vi "dtAppMain.vi"() -> ()   [LabVIEW 2016]
doc: "Top-level application."
uses:
  Typedefs/ContextID.ctl
  ContextIDFactory/ContextIDFactory.lvclass
  ContextThisComponent/ContextThisComponent.lvclass
  home/andres/ct_cmpuserevents/ComponentTemplateCore/ComponentModel/ComponentModel/Context/Context.lvclass
  InvokerThisComponent/InvokerThisComponent.lvclass
  home/andres/ct_cmpuserevents/ComponentTemplateCore/ComponentModel/ComponentModel/Invoker/Invoker.lvclass
  CommandFactory/CommandFactory.lvclass
  StateFactory/StateFactory.lvclass
  home/andres/ct_cmpuserevents/IStateFactory/IStateFactory.lvclass
  Model/Model/Model.lvclass
  home/andres/ct_cmpuserevents/IModel/IModel.lvclass
  PubSubDataEvent/PubSubDataEvent.lvclass
  MiddlewareSALThisComponent/MiddlewareSALThisComponent.lvclass
  home/andres/ct_cmpuserevents/ComponentTemplateCore/ComponentModel/ComponentModel/Middleware/Middleware.lvclass
  MiddlewareSALThisComponent/ProgrammaticInitialization/ProgrammaticInitialization.lvclass
  ComponentTemplateCore/ComponentModel/ComponentModel/UserEventBasedController/UserEventBasedController.lvclass
  home/andres/ct_cmpuserevents/ComponentTemplateCore/ComponentModel/ComponentModel/Controller/Controller.lvclass
  Typedefs/CommandValue.ctl
  ComponentTemplateCore/ComponentModel/ComponentModelRT/LoopTimer/LoopTimer/LoopTimer.lvclass
  home/andres/ct_cmpuserevents/ComponentTemplateCore/ComponentModel/ComponentModelRT/LoopTimer/ILoopTimer/ILoopTimer.lvclass
  ComponentTemplateCore/ComponentModel/ComponentModel/DTTLListener/DTTLListener.lvclass
  home/andres/ct_cmpuserevents/ComponentTemplateCore/ComponentModel/ComponentModel/TimedLoopListener/TimedLoopListener.lvclass
  Model/Target/WindowsTarget/WindowsTarget.lvclass
  home/andres/ct_cmpuserevents/Model/Target/Target/Target.lvclass
  ComponentTemplateCore/ComponentModel/ComponentModel/Heartbeat/Heartbeat/Heartbeat.lvclass
  home/andres/ct_cmpuserevents/ComponentTemplateCore/ComponentModel/ComponentModel/Heartbeat/IHeartbeat/IHeartbeat.lvclass
  ComponentTemplateCore/ComponentModel/ComponentModel/Rendezvous/Rendezvous.lvclass
  ComponentTemplateCore/ComponentModel/ComponentModel/CommandEvent/CommandEvent.lvclass
  ComponentTemplateCore/ComponentModel/ComponentModel/MiddlewareProcessEvent/MiddlewareProcessEvent.lvclass
  Model/Model/Model.lvclass/Model.ctl
  Typedefs/StateValue.ctl
  ts_sallv_exa/DataTypes/logevent_SummaryState.ctl
  ComponentTemplateCore/ComponentModel/ComponentModel/UserEventBasedController/UserEventBasedController.lvclass/UserEventBasedController.ctl
  ComponentTemplateCore/ComponentModel/ComponentModel/Middleware/Middleware.lvclass/Middleware.ctl
  ComponentTemplateCore/Application/AppDT/AppDT.lvclass
  ComponentTemplateCore/Application/AppDT/AppDT.lvclass/AppDT.ctl
  Typedefs/EXATypedefs.lvlib
  ComponentTemplateCore/ComponentModel/ComponentModel/Middleware/Middleware.lvclass
  ts_sallv_exa/SALLV_EXA.lvlib
  ComponentTemplateCore/ComponentModel/ComponentModel/ConfigurationFileReader/ConfigurationFileReader.lvclass
panel:
  out "error out":errorcluster
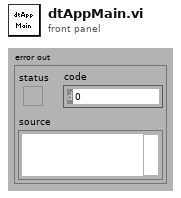
[diagram p1: front panel]
types:
  T1 = typedef "EXATypedefs.lvlib/ContextID.ctl" = enum16{"ExA"}
  T2 = typedef "EXATypedefs.lvlib/CommandValue.ctl" = enum16{"Disable", "Enable", "Exit", "GoToStandby", "OnHeartbeat", "OnIncomingMessagingError", "OnInterrupt", "Start"}
  T3 = typedef "SALLV_EXA.lvlib/logevent_SummaryState.ctl" = cluster{"summaryState":enum16{"", " OfflineState", "StandbyState", "DisabledState", "EnabledState", "FaultState"}, "priority":i32}
  T4 = typedef "EXATypedefs.lvlib/StateValue.ctl" = enum16{"", " DisabledState", "EnabledState", "FaultState", "OfflineState", "StandbyState"}
  T5 = typedef "ConfigurationTypedefs.lvlib/SALVisSettings.ctl" = cluster{"Subsystem":string, "SAL Vis Path":path, "Events":T6, "Telemetry":T7, "Commands":T8}
  T6 = typedef "ProgrammaticInitialization.lvclass/evntsToSubscribeView.ctl" = string[]
  T7 = typedef "ProgrammaticInitialization.lvclass/tlmtryToSubscribeView.ctl" = string[]
  T8 = typedef "ProgrammaticInitialization.lvclass/cmdsToSubscribeDL.ctl" = string[]
  T9 = enum32{"invalid app kind", "Development System", "Run Time System", "Student Edition", "Embedded LabVIEW", "Evaluation", "Custom"}
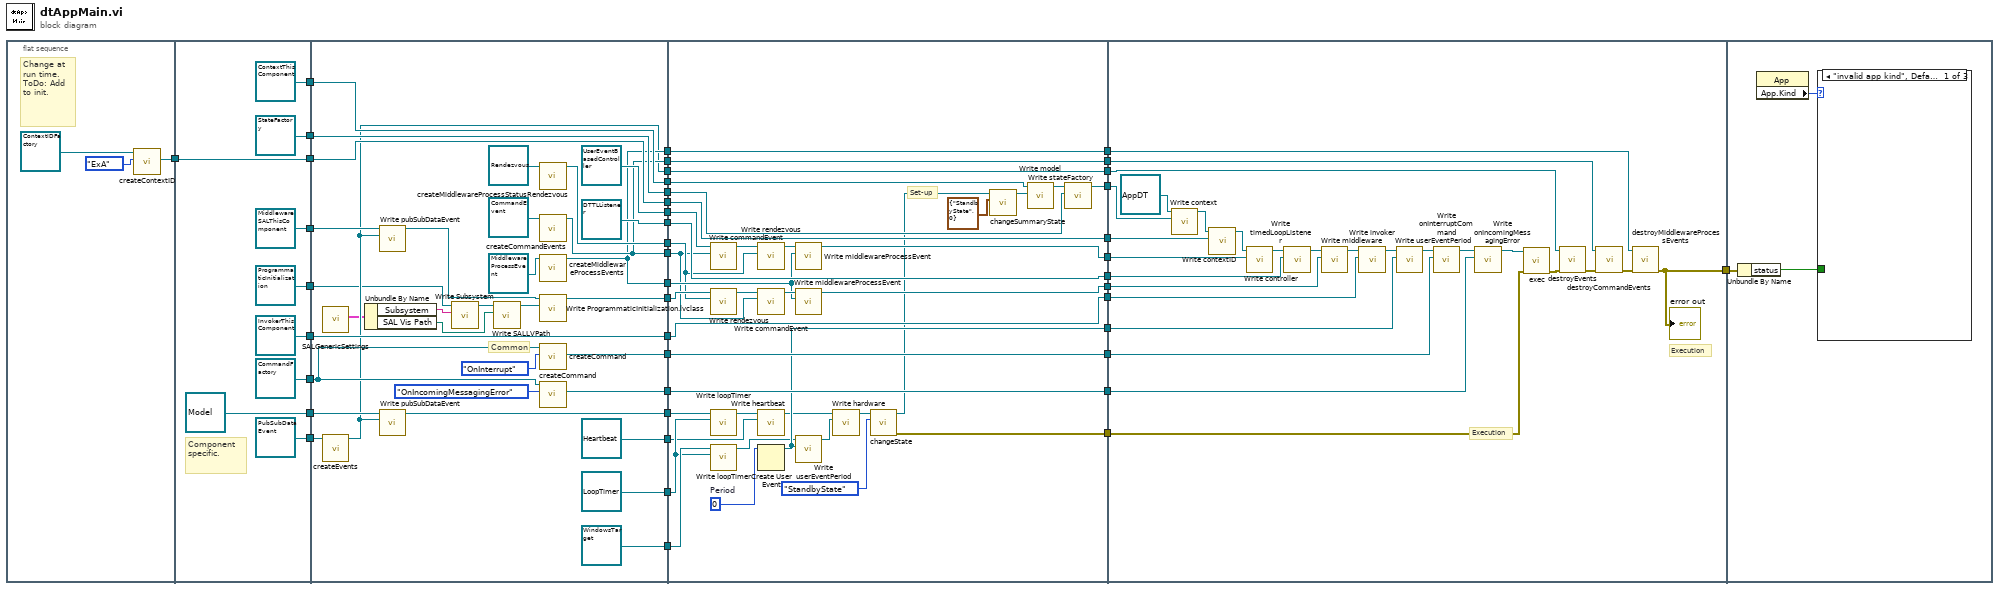
[diagram p0: block diagram]
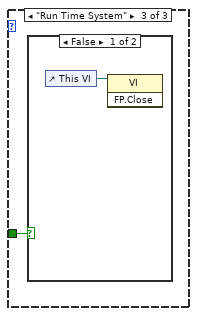
[diagram p3: hidden frame]
diagram:
  n1 = flat-sequence {
    tunnel: [w45] -> w36
    tunnel: [w53] -> w39
    tunnel: [refnum<class "ContextThisComponent.lvclass"> refnum ("ConcreteContext.lvlib:ConcreteContext1.lvclass")] -> w38
    tunnel: [refnum<class "InvokerThisComponent.lvclass"> refnum ("InvokerThisComponent.lvclass")] -> w37
    tunnel: w36 -> [w53]
    tunnel: [refnum<class "CommandFactory.lvclass"> refnum ("CommandFactory.lvclass")] -> w27
    tunnel: [refnum<class "StateFactory.lvclass"> refnum ("ConcreteStateFactory.lvlib:ConcreteStateFactory.lvclass")] -> w25
    tunnel: [refnum<class "Model.lvclass"> refnum ("ConcreteModel.lvclass")] -> w23
    tunnel: [refnum<class "MiddlewareSALThisComponent.lvclass"> refnum ("MiddlewareSALThisComponent.lvclass")] -> w14
    tunnel: [refnum<class "PubSubDataEvent.lvclass"> refnum ("pubSubDataEvent")] -> w13
    tunnel: [refnum<class "ProgrammaticInitialization.lvclass"> refnum ("ProgrammaticInitialization.lvclass")] -> w1
    tunnel: [w87] -> w43
    tunnel: [w86] -> w42
    tunnel: [refnum<class "UserEventBasedController.lvclass"> refnum ("UserEventBasedController in")] -> w41
    tunnel: [w85] -> w40
    tunnel: w39 -> [w87]
    tunnel: w38 -> [w86]
    tunnel: w37 -> [w85]
    tunnel: [refnum<class "DTTLListener.lvclass"> refnum ("DTTLListener.lvclass")] -> w30
    tunnel: [w84] -> w28
    tunnel: w27 -> [w80]
    tunnel: [w83] -> w26
    tunnel: w25 -> [w83]
    tunnel: [w66] -> w24
    tunnel: w23 -> [w67]
    tunnel: [refnum<class "LoopTimer.lvclass"> refnum ("ComponentModelRT.lvlib:LoopTimer.lvclass")] -> w22
    tunnel: [w78] -> w19
    tunnel: [refnum<class "WindowsTarget.lvclass"> refnum ("WindowsTarget.lvclass")] -> w17
    tunnel: [refnum<class "Heartbeat.lvclass"> refnum ("Heartbeat.lvclass")] -> w15
    tunnel: w14 -> [w65]
    tunnel: w13 -> [w74]
    tunnel: [w62] -> w12
    tunnel: [w70] -> w11
    tunnel: [w69] -> w10
    tunnel: [w68] -> w9
    tunnel: [w64] -> w6
    tunnel: [w69] -> w4
    tunnel: [w68] -> w2
    tunnel: w1 -> [w61]
    tunnel: w43 -> [w127]
    tunnel: w42 -> [w120]
    tunnel: w41 -> [w101]
    tunnel: w40 -> [w126]
    tunnel: [w127] -> w35
    tunnel: [w126] -> w34
    tunnel: [w97] -> w33
    tunnel: [w114] -> w32
    tunnel: [w125] -> w31
    tunnel: w30 -> [w125]
    tunnel: [w124] -> w29
    tunnel: w28 -> [w124]
    tunnel: w26 -> [w122]
    tunnel: w24 -> [w116]
    tunnel: w22 -> [w111]
    tunnel: [w121] -> w21
    tunnel: [w119] -> w20
    tunnel: w19 -> [w119]
    tunnel: [w90] -> w18
    tunnel: w17 -> [w115]
    tunnel: w15 -> [w108]
    tunnel: w12 -> [w107]
    tunnel: w11 -> [w102]
    tunnel: w10 -> [w100]
    tunnel: w9 -> [w103]
    tunnel: [w92] -> w8
    tunnel: [w96] -> w7
    tunnel: w6 -> [w96]
    tunnel: [w95] -> w5
    tunnel: w4 -> [w95]
    tunnel: [w94] -> w3
    tunnel: w2 -> [w94]
    tunnel: w31 -> [w149]
    tunnel: w32 -> [w147]
    tunnel: w33 -> [w151]
    tunnel: w34 -> [w148]
    tunnel: w35 -> [w153]
    tunnel: w29 -> [w145]
    tunnel: w21 -> [w144]
    tunnel: w20 -> [w142]
    tunnel: w18 -> [w141]
    tunnel: [w129] -> w16
    tunnel: w8 -> [w136]
    tunnel: w7 -> [w135]
    tunnel: w5 -> [w134]
    tunnel: w3 -> [w133]
    tunnel: w16 -> [w155]
    frame #0 {
      # "Change at run time.\nToDo: Add to init."
      n2 = call-dynamic "createContextID.vi"("ContextID"=ContextID."ExA", "ContextIDFactory in"=refnum<class "ContextIDFactory.lvclass"> refnum) -> ("contextID"=w45:refnum<class "ContextID.lvclass">)  [unwired: 7 in, 2 out]
    }
    frame #1 {
      # "Component specific."
    }
    frame #2 {
      # "Common"
      n3 = call "SALGenericSettings.vi"() -> ("Generic SAL Definitions"=w58:T5)  [unwired: 9 in, 2 out]
      n4 = call "createEvents.vi"("PubSubDataEvent in"=w74) -> ("PubSubDataEvent out"=w64:refnum<class "PubSubDataEvent.lvclass">)  [unwired: 9 in, 1 out]
      n5 = Unbundle By Name(w58) -> ("Subsystem"=w56:string, "SAL Vis Path"=w57:path)
      n6 = call "Write pubSubDataEvent.vi"("pubSubDataEvent in"=w64, "MiddlewareSALThisComponent.lvclass in"=w65) -> ("MiddlewareSALThisComponent.lvclass out"=w63:refnum<class "MiddlewareSALThisComponent.lvclass">)  [unwired: 9 in]
      n7 = call "Write pubSubDataEvent.vi"("PubSubDataEvent.lvclass"=w64, "Model in"=w67) -> ("Model out"=w66:refnum<class "Model.lvclass">)  [unwired: 9 in]
      n8 = call-dynamic "Write Subsystem.vi"("Subsystem"=w56, "ProgrammaticInitialization in"=w61) -> ("ProgrammaticInitialization out"=w60:refnum<class "ProgrammaticInitialization.lvclass">)  [unwired: 8 in, 1 out]
      n9 = call-dynamic "Write SALLVPath.vi"("SALLVPath"=w57, "ProgrammaticInitialization in"=w60) -> ("ProgrammaticInitialization out"=w59:refnum<class "ProgrammaticInitialization.lvclass">)  [unwired: 8 in, 1 out]
      n10 = call "createMiddlewareProcessStatusRendezvous.vi"("Rendezvous in"=refnum<class "Rendezvous.lvclass"> refnum ("rendezvous")) -> ("Rendezvous out"=w70:refnum<class "Rendezvous.lvclass">)  [unwired: 9 in, 1 out]
      n11 = call "createCommandEvents.vi"("CommandEvent in"=refnum<class "CommandEvent.lvclass"> refnum ("commandEvent")) -> ("CommandEvent out"=w69:refnum<class "CommandEvent.lvclass">)  [unwired: 9 in, 1 out]
      n12 = call "createMiddlewareProcessEvents.vi"("MiddlewareProcessEvent in"=refnum<class "MiddlewareProcessEvent.lvclass"> refnum ("middlewareProcessEvent")) -> ("MiddlewareProcessEvent out"=w68:refnum<class "MiddlewareProcessEvent.lvclass">)  [unwired: 9 in, 1 out]
      n13 = call-dynamic "Write ProgrammaticInitialization.lvclass.vi"("ProgrammaticInitialization.lvclass"=w59, "MiddlewareSALThisComponent in"=w63) -> ("MiddlewareSALThisComponent out"=w62:refnum<class "MiddlewareSALThisComponent.lvclass">)  [unwired: 8 in, 1 out]
      n14 = call-dynamic "createCommand.vi"("commandValue"=CommandValue."OnInterrupt", "CommandFactory in"=w80) -> ("command"=w84:refnum<class "Command.lvclass">)  [unwired: 7 in, 2 out]
      n15 = call-dynamic "createCommand.vi"("commandValue"=CommandValue."OnIncomingMessagingError", "CommandFactory in"=w80) -> ("command"=w78:refnum<class "Command.lvclass">)  [unwired: 7 in, 2 out]
    }
    frame #3 {
      w117 = i64 0  # Period
      # "Set-up"
      n16 = call "Write commandEvent.vi"("commandEvent"=w100, "UserEventBasedController in"=w101) -> ("UserEventBasedController out"=w99:refnum<class "UserEventBasedController.lvclass">)  [unwired: 9 in]
      n17 = call "Write rendezvous.vi"("Rendezvous.lvclass"=w102, "Middleware in"=w107) -> ("Middleware out"=w106:refnum<class "MiddlewareSALThisComponent.lvclass">)  [unwired: 9 in]
      n18 = call "Write loopTimer.vi"("LoopTimer.lvclass"=w111, "Model in"=w116) -> ("Model out"=w110:refnum<class "Model.lvclass">)  [unwired: 9 in]
      n19 = call "Write loopTimer.vi"("ILoopTimer.lvclass"=w111, "WindowsTarget in"=w115) -> ("WindowsTarget out"=w113:refnum<class "WindowsTarget.lvclass">)  [unwired: 8 in, 1 out]
      n20 = call "Write rendezvous.vi"("rendezvous"=w102, "UserEventBasedController in"=w99) -> ("UserEventBasedController out"=w98:refnum<class "UserEventBasedController.lvclass">)  [unwired: 9 in]
      n21 = call "Write commandEvent.vi"("CommandEvent.lvclass"=w100, "Middleware in"=w106) -> ("Middleware out"=w105:refnum<class "MiddlewareSALThisComponent.lvclass">)  [unwired: 9 in]
      n22 = call "Write heartbeat.vi"("IHeartbeat.lvclass"=w108, "Model in"=w110) -> ("Model out"=w109:refnum<class "Model.lvclass">)  [unwired: 9 in]
      n23 = Create User Event(user event datatype=w117) -> (user event=w114:refnum<user-event>)  [unwired: 1 in, 1 out]
      n24 = call "Write middlewareProcessEvent.vi"("middlewareProcessEvent"=w103, "UserEventBasedController in"=w98) -> ("UserEventBasedController out"=w97:refnum<class "UserEventBasedController.lvclass">)  [unwired: 9 in]
      n25 = call "Write middlewareProcessEvent.vi"("middlewareProcessEvent"=w103, "Middleware in"=w105) -> ("Middleware out"=w92:refnum<class "MiddlewareSALThisComponent.lvclass">)  [unwired: 9 in]
      n26 = call "Write userEventPeriod.vi"("userEventPeriod"=w114, "WindowsTarget in"=w113) -> ("WindowsTarget out"=w104:refnum<class "WindowsTarget.lvclass">)  [unwired: 8 in, 1 out]
      n27 = call "Write hardware.vi"("Hardware.lvclass"=w104, "Model in"=w109) -> ("Model out"=w93:refnum<class "Model.lvclass">)  [unwired: 8 in, 1 out]
      n28 = call-dynamic "changeState.vi"("newState"=StateValue."StandbyState" ("StateValue"), "Model in"=w93) -> ("error out"=w90:errorcluster, "Model out"=w91:refnum<class "Model.lvclass">)  [unwired: 8 in]
      n29 = call-dynamic "changeSummaryState.vi"("logevent_SummaryState"=T3 {"summaryState"=enum."StandbyState", "priority"=0}, "Model in"=w91) -> ("Model out"=w112:refnum<class "Model.lvclass">)  [unwired: 8 in, 1 out]
      n30 = call-dynamic "Write model.vi"("Model.lvlib:Model.lvclass"=w112, "ConcreteContext1 in"=w120) -> ("ConcreteContext1 out"=w123:refnum<class "ContextThisComponent.lvclass">)  [unwired: 9 in]
      n31 = call-dynamic "Write stateFactory.vi"("StateFactory.lvlib:StateFactory.lvclass"=w122, "ConcreteContext1 in"=w123) -> ("ConcreteContext1 out"=w121:refnum<class "ContextThisComponent.lvclass">)  [unwired: 9 in]
    }
    frame #4 {
      # "Execution"
      # "Execution"
      n32 = call "Write context.vi"("context"=w144, "AppDT in"=refnum<class "AppDT.lvclass"> refnum ("AppRT9074 in")) -> ("AppDT out"=w154:refnum<class "AppDT.lvclass">)  [unwired: 8 in, 1 out]
      n33 = call "Write contextID.vi"("contextID"=w153, "AppDT in"=w154) -> ("AppDT out"=w152:refnum<class "AppDT.lvclass">)  [unwired: 8 in, 1 out]
      n34 = call "Write controller.vi"("controller"=w151, "AppDT in"=w152) -> ("AppDT out"=w150:refnum<class "AppDT.lvclass">)  [unwired: 8 in, 1 out]
      n35 = call "Write timedLoopListener.vi"("TimedLoopListener.lvclass"=w149, "AppDT in"=w150) -> ("AppDT out"=w138:refnum<class "AppDT.lvclass">)  [unwired: 8 in, 1 out]
      n36 = call "Write middleware.vi"("middleware"=w136, "AppDT in"=w138) -> ("AppDT out"=w137:refnum<class "AppDT.lvclass">)  [unwired: 9 in]
      n37 = call "Write invoker.vi"("invoker"=w148, "AppDT in"=w137) -> ("AppDT out"=w140:refnum<class "AppDT.lvclass">)  [unwired: 8 in, 1 out]
      n38 = call "Write userEventPeriod.vi"("userEventPeriod"=w147, "AppDT in"=w140) -> ("AppDT out"=w146:refnum<class "AppDT.lvclass">)  [unwired: 8 in, 1 out]
      n39 = call "Write onInterruptCommand.vi"("onInterruptCommand"=w145, "AppDT in"=w146) -> ("AppDT out"=w143:refnum<class "AppDT.lvclass">)  [unwired: 8 in, 1 out]
      n40 = call "Write onIncomingMessagingError.vi"("Command.lvclass"=w142, "AppDT in"=w143) -> ("AppDT out"=w139:refnum<class "AppDT.lvclass">)  [unwired: 8 in, 1 out]
      n41 = call-dynamic "exec.vi"("error in (no error)"=w141, "AppDT in"=w139) -> ("error out"=w132:errorcluster)  [unwired: 8 in, 1 out]
      n42 = call "destroyEvents.vi"("error in (no error)"=w132, "PubSubDataEvent in"=w135) -> ("error out"=w131:errorcluster)  [unwired: 8 in, 1 out]
      n43 = call "destroyCommandEvents.vi"("error in (no error)"=w131, "CommandEvent in"=w134) -> ("error out"=w130:errorcluster)  [unwired: 8 in, 1 out]
      n44 = call "destroyMiddlewareProcessEvents.vi"("error in (no error)"=w130, "MiddlewareProcessEvent in"=w133) -> ("error out"=w129:errorcluster)  [unwired: 8 in, 1 out]
      "error out" <- w129
    }
    frame #5 {
      n45 = Unbundle By Name(w155) -> ("status"=w156:bool)
      n46 = property class="App"() -> ("App.Kind"=w157:T9)  [unwired: 2 in, 2 out]
      n47 = case shown="\"invalid app kind\", Default" w157 {
        tunnel: w156 -> [_ _ w158]
        frame "invalid app kind", Default {
        }
        frame "Development System" {
        }
        frame "Run Time System" {
          n48 = case shown="False" w158 {
            frame False {
              n49 = control-ref of="This VI"() -> (w159:refnum<vi>)
              n50 = invoke class="VI" method="FP.Close"(reference=w159) -> ()  [unwired: 2 in, 3 out]
            }
            frame True {
            }
          }
        }
      }
    }
  }
